vi "Test Load Waveform from TDMS.vi"(8 "error in (no error)":errorcluster) -> (0 "error out":errorcluster)   [LabVIEW 2016]
uses:
  <vilib>/addons/_JKI Toolkits/Caraya/classes/Assert/Assert True.vi
  <vilib>/addons/_JKI Toolkits/Caraya/classes/Assert/Assert Less Or Equal_Variant.vi
  <vilib>/addons/_JKI Toolkits/Caraya/classes/Assert/Assert Almost Equal_Float.vi
  <vilib>/addons/_JKI Toolkits/Caraya/classes/Assert/Assert False.vi
  <vilib>/addons/_JKI Toolkits/Caraya/classes/Assert/Assert Greater_Variant.vi
  <vilib>/addons/_JKI Toolkits/Caraya/classes/Assert/Assert Greater Or Equal_Variant.vi
  <instrlib>/niRFSGPlayback/niRFSGPlayback Download User Waveform (CSG).vi
  <vilib>/addons/_JKI Toolkits/Caraya/classes/Assert/Assert Equal Value_Variant.vi
  <vilib>/Utility/config.llb/Read Key (Boolean).vi
  Source/SG/SG.lvlib
  <vilib>/addons/_JKI Toolkits/Caraya/classes/Test/Test.lvclass
  <vilib>/addons/_JKI Toolkits/Caraya/classes/Assert/Assert.lvclass
  <vilib>/Utility/config.llb/NI_LVConfig.lvlib
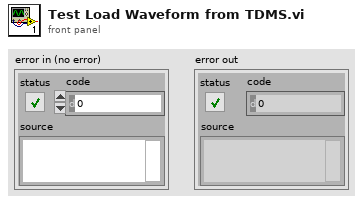
[diagram p1: front panel]
types:
  T1 = enum16{"Waveform.dx greater than 0", "Waveform.y not empty", "Waveform.dx equal to 1/fs", "Sample rate greater than 0", "Signal bandwidth geq to 0", "Burst length greater than 0", "Papr geq to 0", "Start locations not empty", "Stop locations not empty", "Runtime scaling leq to 0", "Entire waveform read", "Papr agrees with playback library calculation", "Idle duration present calculated correctly", "Waveform read from library matches loaded type"}
  T2 = typedef "SG.lvlib/Waveform.ctl" = cluster{"Waveform Name":string, "Waveform":cluster{"x0":dbl, "dx":dbl, "y":csg[]}, "Signal Bandwidth (Hz)":dbl, "PAPR (dB)":dbl, "Burst Length (s)":dbl, "Sample Rate":dbl, "Burst Start Locations":i32[], "Burst Stop Locations":i32[], "Idle Duration Present?":bool, "Runtime Scaling":dbl}
  T3 = typedef "NI_LVConfig.lvlib/Config Data RefNum.ctl" = refnum<k1>
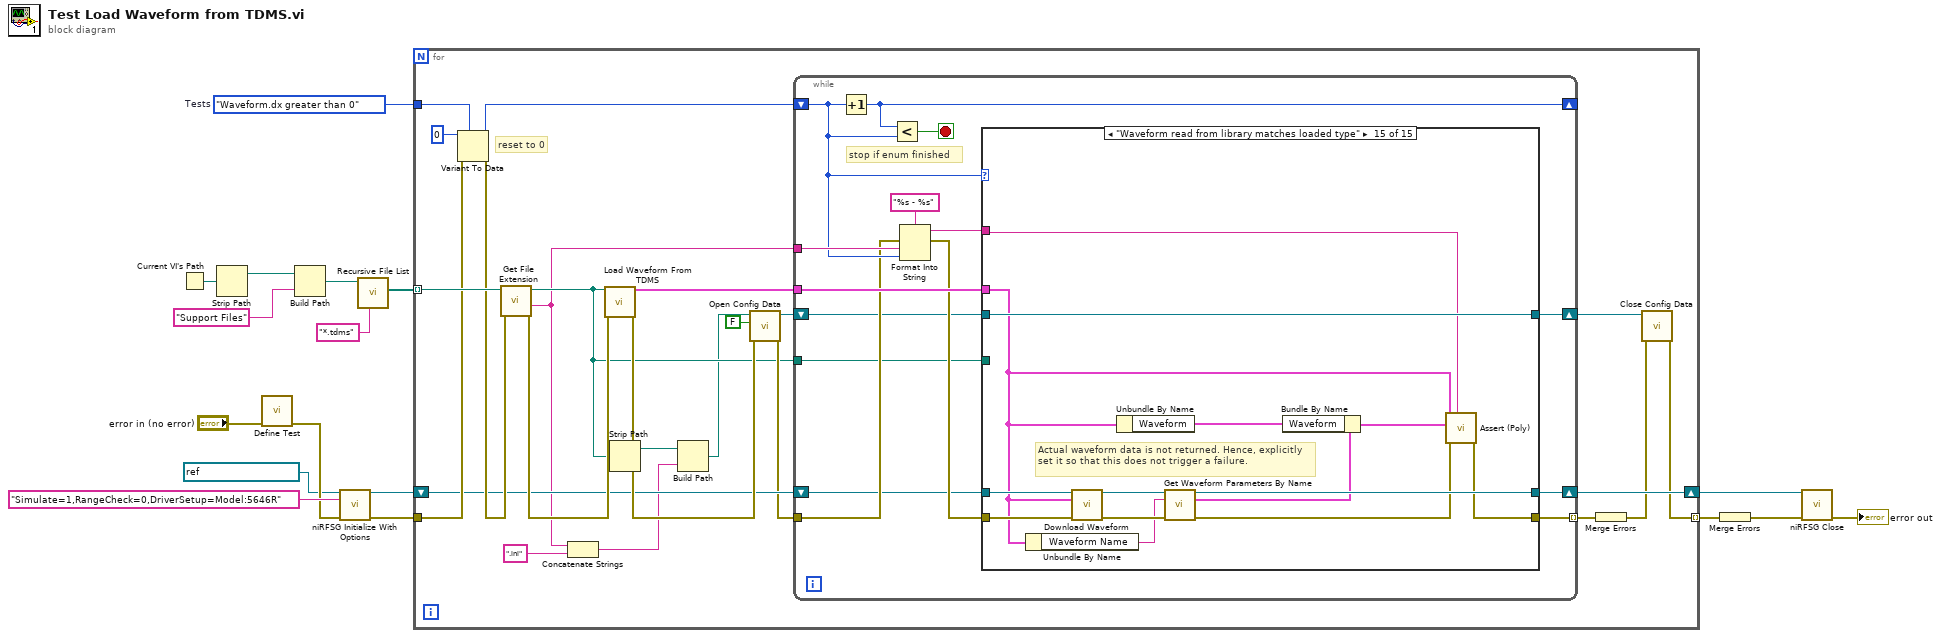
[diagram p0: block diagram]
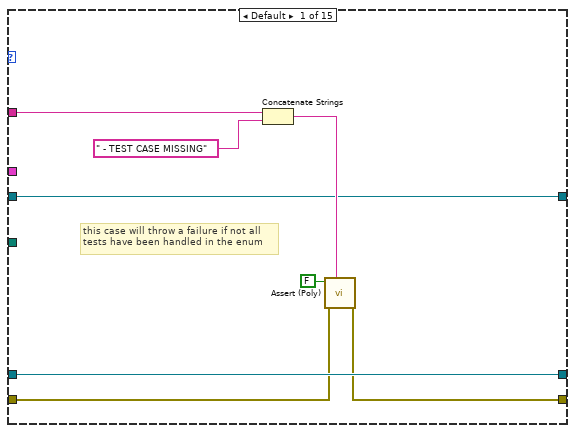
[diagram p2: hidden frame]
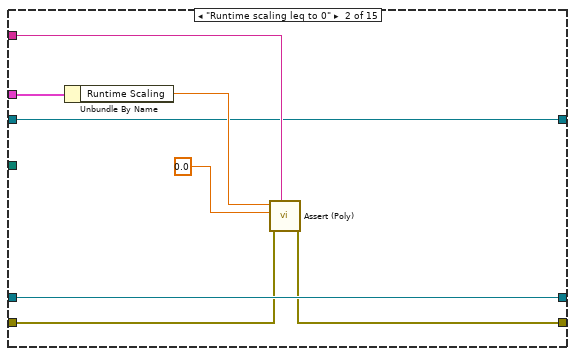
[diagram p3: hidden frame]
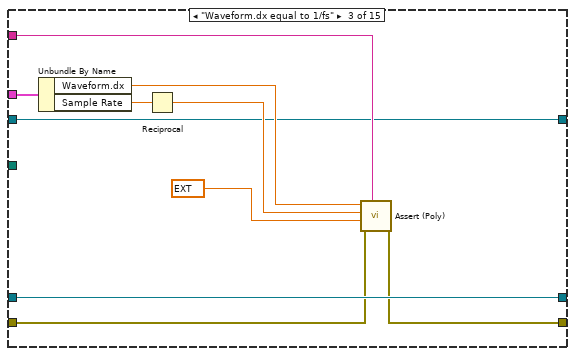
[diagram p4: hidden frame]
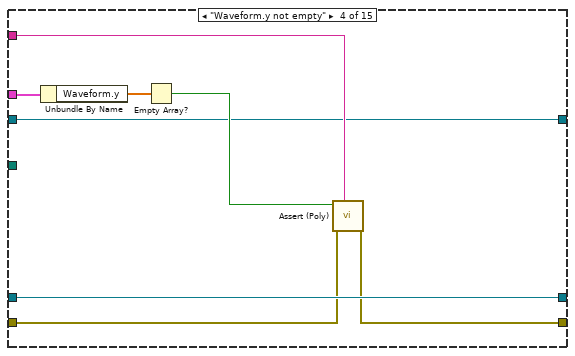
[diagram p5: hidden frame]
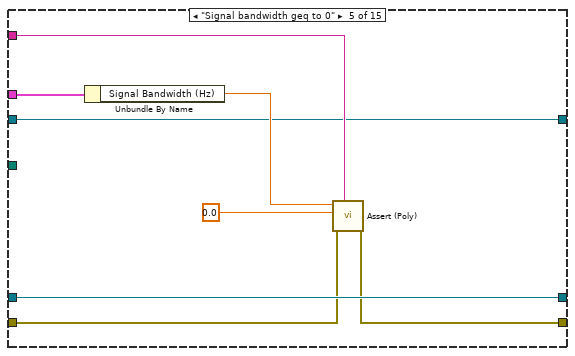
[diagram p6: hidden frame]
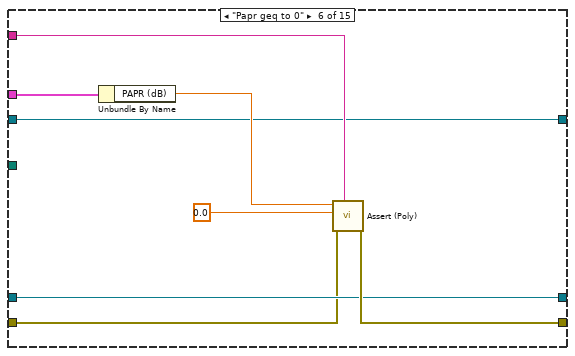
[diagram p7: hidden frame]
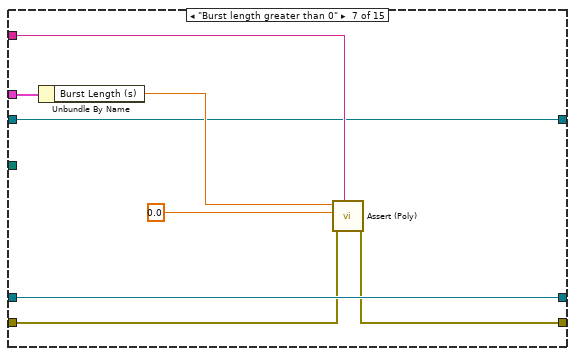
[diagram p8: hidden frame]
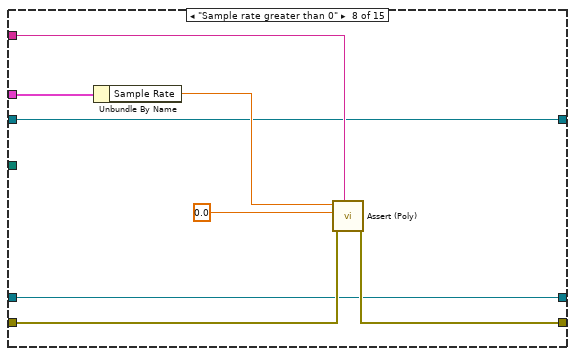
[diagram p9: hidden frame]
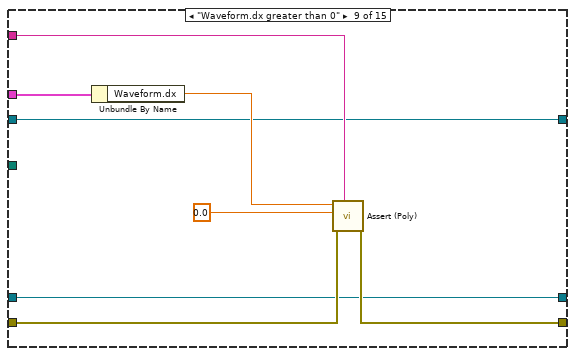
[diagram p10: hidden frame]
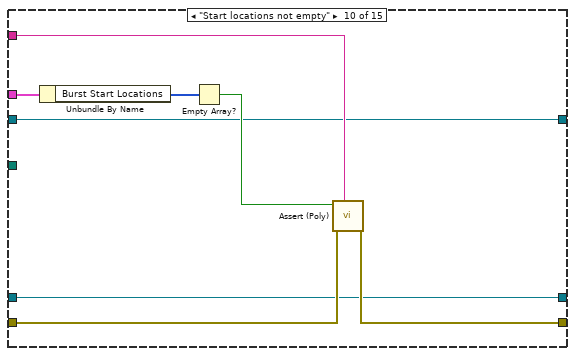
[diagram p11: hidden frame]
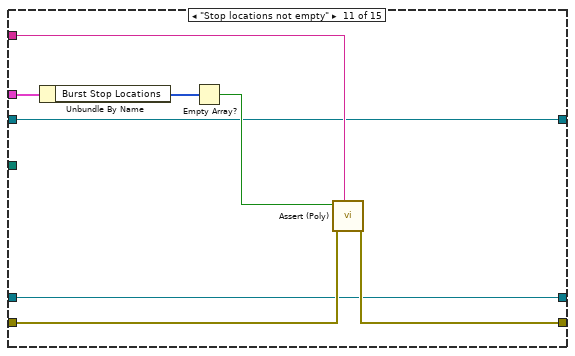
[diagram p12: hidden frame]
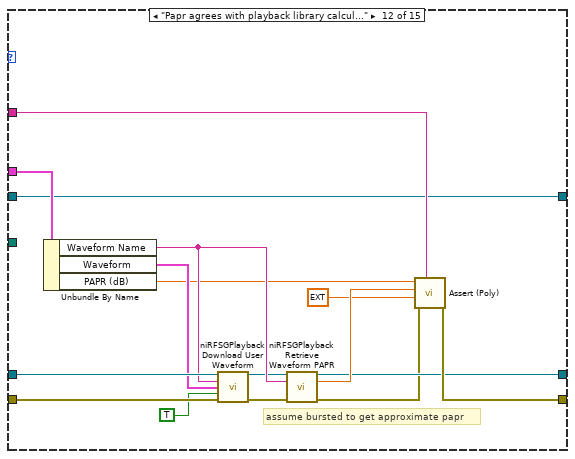
[diagram p13: hidden frame]
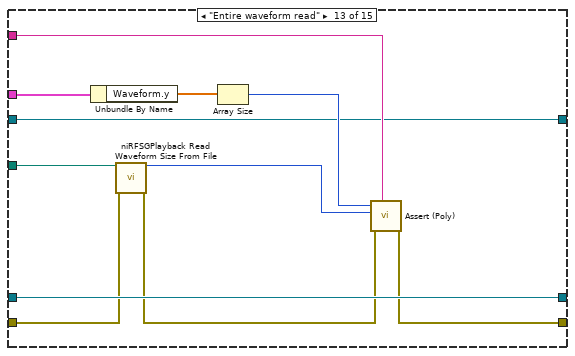
[diagram p14: hidden frame]
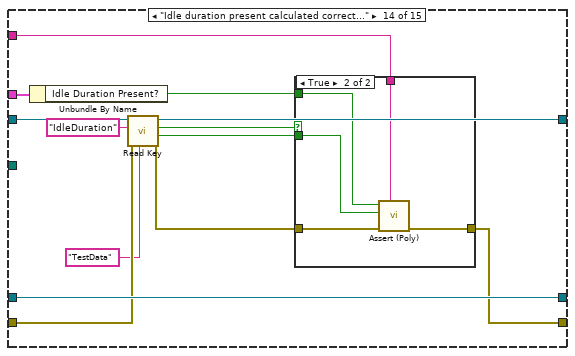
[diagram p15: hidden frame]
diagram:
  w9 = T1."Waveform.dx greater than 0"  # Tests
  n1 = Current VI's Path() -> (path=w17:path)
  n2 = Strip Path(path=w17) -> (stripped path=w16:path)  [unwired: 1 out]
  n3 = call <vilib>:"Define Test.vi"("error in (no error)"="error in (no error)") -> ("error out"=w6:errorcluster)  [unwired: 10 in]
  n4 = Build Path(base path=w16, name or relative path="Support Files") -> (appended path=w12:path)
  n5 = call <instrlib>:"niRFSG Initialize With Options.vi"("resource name"=refnum<k15> "SimulatedDevice", "option string"="Simulate=1,RangeCheck=0,DriverSetup=Model:5646R", "error in"=w6) -> ("instrument handle"=w7:refnum<k15>, "error out"=w5:errorcluster)  [unwired: 11 in]
  n6 = call <vilib>:"Recursive File List.vi"("pattern"="*.tdms", "Folder Path"=w12) -> ("All Files in Dir"=w11:path[])  [unwired: 5 in, 4 out]
  n7 = for {
    tunnel: w11 -> [w38] mode=indexing
    tunnel: w5 -> [w33]
    tunnel: [w18] -> w10 mode=indexing
    tunnel: w9 -> [w36]
    shift-right: [w30] -> w2
    shift-left: w7 -> [w31]
    # "reset to 0"
    n8 = Variant To Data(error in=w33, type=w36, Variant=i16 0) -> (data=w34:T1, error out=w32:errorcluster)
    n9 = call <vilib>:"Get File Extension.vi"("error in (no error)"=w32, "file"=w38) -> ("error out"=w37:errorcluster, "filename without extension"=w23:string, "dup file"=w26:path)  [unwired: 5 in, 2 out]
    n10 = Concatenate Strings(w23, ".ini" ("string")) -> (w24:string)
    n11 = call "Load Waveform From TDMS.vi"("TDMS File Path"=w26, "error in (no error)"=w37) -> ("Waveform"=w40:T2, "error out"=w41:errorcluster)  [unwired: 12 in]
    n12 = Strip Path(path=w26) -> (stripped path=w25:path)  [unwired: 1 out]
    n13 = Build Path(base path=w25, name or relative path=w24) -> (appended path=w21:path)
    n14 = call <vilib>:"Open Config Data.vi"("error in (no error)"=w41, "create file if necessary (T)"=FALSE, "configuration file path"=w21) -> ("error out"=w27:errorcluster, "refnum"=w29:T3)  [unwired: 6 in, 1 out]
    n15 = while {
      tunnel: w40 -> [w56]
      tunnel: [w43] -> w39 mode=indexing
      tunnel: w23 -> [w54]
      shift-right: [w52] -> _
      shift-left: w34 -> [w51]
      tunnel: w27 -> [w49]
      shift-right: [w47] -> w30
      shift-left: w31 -> [w48]
      tunnel: w26 -> [w46]
      shift-right: [w42] -> w20
      shift-left: w29 -> [w44]
      stop <- w45 stop-if-true
      # "stop if enum finished"
      n16 = Increment(x=w51) -> (x+1=w52:T1)
      n17 = Less?(x=w52, y=w51) -> (x < y?=w45:bool)
      n18 = Format Into String(format string="%s - %s", error in=w49, w54, w51) -> (resulting string=w53:string, error out=w50:errorcluster)  [unwired: 1 in]
      n19 = case shown="\"Waveform read from library matches loaded type\"" w51 {
        tunnel: [w57 w65 w73 w83 w91 w106 w107 w122 w130 w138 w146 w158 w169 w179 w193] -> w43
        tunnel: w56 -> [_ w72 w82 w90 w98 w105 w114 w121 w129 w137 w145 w161 w167 w175 w196]
        tunnel: w53 -> [w62 w69 w77 w87 w95 w102 w111 w118 w126 w134 w142 w154 w168 w178 w195]
        tunnel: w50 -> [w58 w66 w74 w84 w92 w99 w108 w117 w125 w133 w141 w153 w171 w183 w204]
        tunnel: w48 -> [w64 w68 w76 w86 w94 w101 w110 w116 w124 w132 w140 w162 w173 w186 w205]
        tunnel: [w64 w68 w76 w86 w94 w101 w110 w116 w124 w132 w140 w155 w173 w186 w201] -> w47
        tunnel: w46 -> [_ _ _ _ _ _ _ _ _ _ _ _ w172 _ _]
        tunnel: w44 -> [w59 w67 w75 w85 w93 w100 w109 w115 w123 w131 w139 w150 w163 w185 w206]
        tunnel: [w59 w67 w75 w85 w93 w100 w109 w115 w123 w131 w139 w150 w163 w184 w206] -> w42
        frame Default {
          # "this case will throw a failure if not all\ntests have been handled in the enum"
          n20 = Concatenate Strings(w62, " - TEST CASE MISSING" ("Label")) -> (w60:string)
          n21 = call-poly <vilib>:"Assert (Poly).vi"("Label"=w60, "error in (no error)"=w58, "True?"=FALSE) -> ("error out"=w57:errorcluster)  [unwired: 8 in]
        }
        frame "Runtime scaling leq to 0" {
          n22 = Unbundle By Name(w72) -> ("Runtime Scaling"=w71:dbl)
          n23 = call-poly <vilib>:"Assert (Poly).vi"("Label"=w69, "error in (no error)"=w66, "Y"=0.0 ("Runtime Scaling"), "X"=w71) -> ("error out"=w65:errorcluster)  [unwired: 7 in]
        }
        frame "Waveform.dx equal to 1/fs" {
          n24 = Unbundle By Name(w82) -> ("Waveform.dx"=w81:dbl, "Sample Rate"=w80:dbl)
          n25 = Reciprocal(x=w80) -> (1/x=w79:dbl)
          n26 = call-poly <vilib>:"Assert (Poly).vi"("Label"=w77, "error in (no error)"=w74, "Tolerance"=ext 0.00099999999999999999996, "Y"=w79, "X"=w81) -> ("error out"=w73:errorcluster)  [unwired: 6 in]
        }
        frame "Waveform.y not empty" {
          n27 = Unbundle By Name(w90) -> ("Waveform.y"=w89:csg[])
          n28 = Empty Array?(array=w89) -> (empty?=w88:bool)
          n29 = call-poly <vilib>:"Assert (Poly).vi"("Label"=w87, "error in (no error)"=w84, "False?"=w88) -> ("error out"=w83:errorcluster)  [unwired: 8 in]
        }
        frame "Signal bandwidth geq to 0" {
          n30 = Unbundle By Name(w98) -> ("Signal Bandwidth (Hz)"=w97:dbl)
          n31 = call-poly <vilib>:"Assert (Poly).vi"("Label"=w95, "error in (no error)"=w92, "Y"=0.0 ("Signal Bandwidth (Hz)"), "X"=w97) -> ("error out"=w91:errorcluster)  [unwired: 7 in]
        }
        frame "Papr geq to 0" {
          n32 = Unbundle By Name(w105) -> ("PAPR (dB)"=w104:dbl)
          n33 = call-poly <vilib>:"Assert (Poly).vi"("Label"=w102, "error in (no error)"=w99, "Y"=0.0 ("Signal Bandwidth (Hz)"), "X"=w104) -> ("error out"=w106:errorcluster)  [unwired: 7 in]
        }
        frame "Burst length greater than 0" {
          n34 = Unbundle By Name(w114) -> ("Burst Length (s)"=w113:dbl)
          n35 = call-poly <vilib>:"Assert (Poly).vi"("Label"=w111, "error in (no error)"=w108, "Y"=0.0 ("Signal Bandwidth (Hz)"), "X"=w113) -> ("error out"=w107:errorcluster)  [unwired: 7 in]
        }
        frame "Sample rate greater than 0" {
          n36 = Unbundle By Name(w121) -> ("Sample Rate"=w120:dbl)
          n37 = call-poly <vilib>:"Assert (Poly).vi"("Label"=w118, "error in (no error)"=w117, "Y"=0.0 ("Signal Bandwidth (Hz)"), "X"=w120) -> ("error out"=w122:errorcluster)  [unwired: 7 in]
        }
        frame "Waveform.dx greater than 0" {
          n38 = Unbundle By Name(w129) -> ("Waveform.dx"=w128:dbl)
          n39 = call-poly <vilib>:"Assert (Poly).vi"("Label"=w126, "error in (no error)"=w125, "Y"=0.0 ("Signal Bandwidth (Hz)"), "X"=w128) -> ("error out"=w130:errorcluster)  [unwired: 7 in]
        }
        frame "Start locations not empty" {
          n40 = Unbundle By Name(w137) -> ("Burst Start Locations"=w136:i32[])
          n41 = Empty Array?(array=w136) -> (empty?=w135:bool)
          n42 = call-poly <vilib>:"Assert (Poly).vi"("Label"=w134, "error in (no error)"=w133, "False?"=w135) -> ("error out"=w138:errorcluster)  [unwired: 8 in]
        }
        frame "Stop locations not empty" {
          n43 = Unbundle By Name(w145) -> ("Burst Stop Locations"=w144:i32[])
          n44 = Empty Array?(array=w144) -> (empty?=w143:bool)
          n45 = call-poly <vilib>:"Assert (Poly).vi"("Label"=w142, "error in (no error)"=w141, "False?"=w143) -> ("error out"=w146:errorcluster)  [unwired: 8 in]
        }
        frame "Papr agrees with playback library calculation" {
          # "assume bursted to get approximate papr"
          n46 = Unbundle By Name(w161) -> ("Waveform Name"=w159:string, "Waveform"=w160:cluster{"x0":dbl, "dx":dbl, "y":csg[]}, "PAPR (dB)"=w157:dbl)
          n47 = call-poly <instrlib>:"niRFSGPlayback Download User Waveform.vi"("instrument handle in"=w162, "waveform name"=w159, "waveform in"=w160, "burst present"=TRUE, "error in"=w153) -> ("instrument handle out"=w149:refnum<k15>, "error out"=w148:errorcluster)  [unwired: 9 in]
          n48 = call <instrlib>:"niRFSGPlayback Retrieve Waveform PAPR.vi"("instrument handle in"=w149, "waveform name"=w159, "error in"=w148) -> ("instrument handle out"=w155:refnum<k15>, "PAPR"=w156:dbl, "error out"=w152:errorcluster)  [unwired: 10 in]
          n49 = call-poly <vilib>:"Assert (Poly).vi"("Label"=w154, "error in (no error)"=w152, "Tolerance"=ext 0.1, "Y"=w156, "X"=w157) -> ("error out"=w158:errorcluster)  [unwired: 6 in]
        }
        frame "Entire waveform read" {
          n50 = Unbundle By Name(w167) -> ("Waveform.y"=w166:csg[])
          n51 = call <instrlib>:"niRFSGPlayback Read Waveform Size From File.vi"("file path"=w172, "error in"=w171) -> ("waveform size"=w164:i32, "error out"=w170:errorcluster)  [unwired: 12 in]
          n52 = Array Size(array=w166) -> (size(s)=w165:i32)
          n53 = call-poly <vilib>:"Assert (Poly).vi"("Label"=w168, "error in (no error)"=w170, "Y"=w164, "X"=w165) -> ("error out"=w169:errorcluster)  [unwired: 7 in]
        }
        frame "Idle duration present calculated correctly" {
          n54 = Unbundle By Name(w175) -> ("Idle Duration Present?"=w174:bool)
          n55 = call-poly <vilib>:"Read Key.vi"("section"="TestData", "error in (no error)"=w183, "key"="IdleDuration", "refnum"=w185) -> ("error out"=w182:errorcluster, "value"=w176:bool, "found?"=w177:bool, "refnum out"=w184:T3)  [unwired: 4 in]
          n56 = case shown="True" w177 {
            tunnel: w182 -> [w187 w192]
            tunnel: [w187 w191] -> w179
            tunnel: w178 -> [_ w190]
            tunnel: w176 -> [_ w189]
            tunnel: w174 -> [_ w188]
            frame False {
              # "Don't run test if key not found"
            }
            frame True {
              n57 = call-poly <vilib>:"Assert (Poly).vi"("Label"=w190, "error in (no error)"=w192, "Y"=w189, "X"=w188) -> ("error out"=w191:errorcluster)  [unwired: 7 in]
            }
          }
        }
        frame "Waveform read from library matches loaded type" {
          # "Actual waveform data is not returned. Hence, explicitly set it so that this does not trigger a failure."
          n58 = Unbundle By Name(w196) -> ("Waveform Name"=w200:string)
          n59 = call "Download Waveform.vi"("RFSG handle"=w205, "Waveform In"=w196, "error in (no error)"=w204) -> ("RFSG handle out"=w203:refnum<k15>, "error out"=w202:errorcluster)  [unwired: 11 in]
          n60 = Unbundle By Name(w196) -> ("Waveform"=w198:cluster{"x0":dbl, "dx":dbl, "y":csg[]})
          n61 = call "Get Waveform Parameters By Name.vi"("RFSG handle"=w203, "Waveform Name"=w200, "error in (no error)"=w202) -> ("RFSG handle out"=w201:refnum<k15>, "Waveform"=w199:T2, "error out"=w194:errorcluster)  [unwired: 10 in]
          n62 = Bundle By Name(cluster=w199, "Waveform"=w198) -> (w197:T2)
          n63 = call-poly <vilib>:"Assert (Poly).vi"("Label"=w195, "error in (no error)"=w194, "Y"=w197, "X"=w196) -> ("error out"=w193:errorcluster)  [unwired: 7 in]
        }
      }
    }
    n64 = Merge Errors(w39) -> (w19:errorcluster)
    n65 = call <vilib>:"Close Config Data.vi"("error in (no error)"=w19, "refnum"=w20) -> ("error out"=w18:errorcluster)  [unwired: 8 in, 1 out]
  }
  n66 = Merge Errors(w10) -> (w3:errorcluster)
  n67 = call <instrlib>:"niRFSG Close.vi"("instrument handle"=w2, "error in"=w3) -> ("error out"=→"error out":errorcluster)  [unwired: 13 in]
